vi "LS330_Read_Temp.vi"(8 "error in":errorcluster, 10 "Channel":string(combo)="A", 11 "VISA resource name":refnum<visa-resource-name>) -> (0 "error out":errorcluster, 2 "Temp (K)":dbl, 3 "VISA resource name out":refnum<visa-resource-name>)   [LabVIEW 2021]
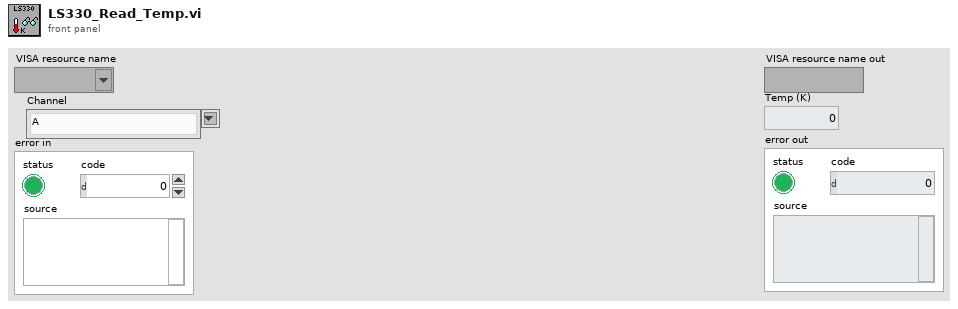
[diagram p1: front panel]
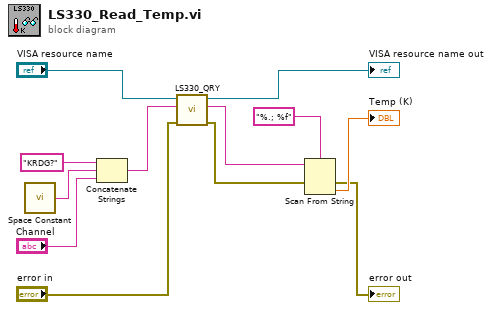
[diagram p0: block diagram]
diagram:
  n1 = call <vilib>:"Space Constant.vi"() -> ("String"=w10:string)
  n2 = Concatenate Strings("KRDG?" ("string"), w10, "Channel") -> (w8:string)
  n3 = call "LS330_QRY.vi"("error in"="error in", "CMD"=w8, "VISA resource name"="VISA resource name") -> ("error out"=w3:errorcluster, "OUT"=w4:string, "VISA resource name out"=→"VISA resource name out":refnum<visa-resource-name>)  [unwired: 5 in, 1 out]
  n4 = Scan From String(format string="%.; %f", input string=w4, error in=w3) -> (error out=→"error out":errorcluster, output 1=→"Temp (K)":dbl)  [unwired: 2 in, 2 out]
